vi "PID360.vi"(10 "Robot":dbl, 11 "Target":dbl) -> (3 "Numeric":dbl)   [LabVIEW 2015]
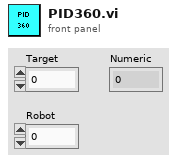
[diagram p1: front panel]
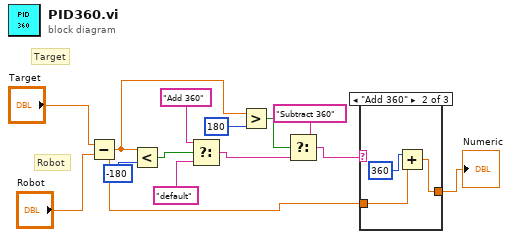
[diagram p0: block diagram]
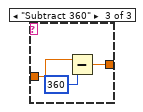
[diagram p3: hidden frame]
diagram:
  # "Robot"
  # "Target"
  n1 = Subtract(x="Target", y="Robot") -> (x-y=w3:dbl)
  n2 = Less?(x=w3, y=-180) -> (x < y?=w6:bool)
  n3 = Select(t="Add 360", s=w6, f="default") -> (s? t:f=w8:string)
  n4 = Greater?(x=w3, y=180) -> (0:w7:bool)
  n5 = Select(t="Subtract 360", s=w7, f=w8) -> (s? t:f=w4:string)
  n6 = case shown="\"Add 360\"" w4 {
    tunnel: w3 -> [w14 w16 w19]
    tunnel: [w14 w15 w18] -> w2
    frame "default", Default {
    }
    frame "Add 360" {
      n7 = Add(x=360, y=w16) -> (x+y=w15:dbl)
    }
    frame "Subtract 360" {
      n8 = Subtract(x=w19, y=360) -> (x-y=w18:dbl)
    }
  }
  "Numeric" <- w2
